vi "Control Reference Disable Mode.vi"(0 "control references in":refnum<vi>[](array[refnum]), 5 "disabled":T1(ring), 11 "error in":errorcluster) -> (15 "error out":errorcluster)   [LabVIEW 2015, in "TLB` Template.lvlib"]
doc: "set UI button display state.\n\n<B>Input Parameters</B>\n\n<B>control references in</B> control references to be operated on.\n\n<B>disabled</B> UI control display state.\n\n<B>Enabled</B>- button is selectable\n<B>Disabled</B>- button is unselecable.\n<B>Disabled and Grayed Out</B>-button is unselecable and grayed out.\n\n<B>error in</B> describes error conditions that occur before this node runs. This input provides standard error in functionality.\n\n<B>Output Parameters</B>\n\n<B>error out</B> contains error information. This output provides standard error out functionality."
uses:
  TLB` Template.lvlib
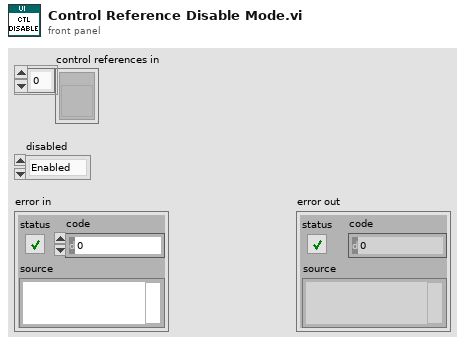
[diagram p1: front panel]
types:
  T1 = enum8{"Enabled", "Disabled", "Disabled and Grayed Out"}
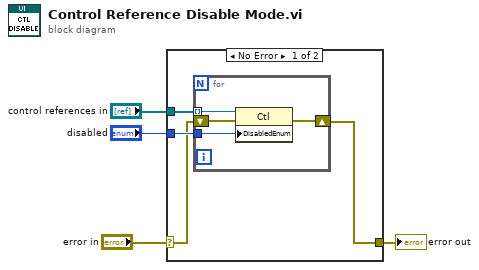
[diagram p0: block diagram]
diagram:
  n1 = case shown="No Error" "error in" {
    selector: "error in" -> [w6 w13]
    tunnel: "disabled" -> [w8 _]
    tunnel: "control references in" -> [w7 _]
    tunnel: [w5 w13] -> w1
    frame No Error {
      n2 = for {
        tunnel: w8 -> [w12]
        tunnel: w7 -> [w11] mode=indexing
        shift-right: [w9] -> w5
        shift-left: w6 -> [w10]
        n3 = property class="Ctl"(reference=w11, error in=w10, "DisabledEnum"=w12) -> (error out=w9:errorcluster)  [unwired: 1 out]
      }
    }
    frame Error {
    }
  }
  "error out" <- w1
